vi "run.create.vi"(6 "Additional Configuration":T1, 8 "error in":errorcluster, 9 "Timing":cluster{"Start":timestamp, "End":timestamp} {"End" format="%<%x %.3X>T"; "Start" format="%<%x %.3X>T"}, 10 "Titles":cluster{"Name":string, "Description":string}, 11 "Nominal Client in":refnum<class "Nominal Client.lvclass">) -> (0 "error out":errorcluster, 2 "Run":refnum<class "Run.lvclass">, 3 "Nominal Client out":refnum<class "Nominal Client.lvclass">, 4 "Response body":string)   [LabVIEW 2020, in "Nominal Client.lvclass"]
doc: "Create a new run in Nominal.\nThrows if start is equal to or after end."
uses:
  Nominal Client.lvclass
  Run/Run.lvclass
  Nominal Client.lvclass/Nominal Client.ctl
  nominal types/workspace/workspace.lvclass/workspace.ctl
  workspace.get.vi
  <vilib>/JDP Science/JSONtext/Merge into Object.vi
  workspace.add_to_payload.vi/88650e10-de3e-481c-85db-71cb0fdf4485.vi
  nominal types/workspace/rid.get.vi
  <vilib>/LabVIEW Open Source Project/Epoch Date & Time/epoch.UNIX/Epoch.UNIX.lvclass
  C:/Program Files (x86)/National Instruments/LabVIEW 2020/vi.lib/LabVIEW Open Source Project/Epoch Date & Time/epoch/Epoch.lvclass
  <vilib>/LabVIEW Open Source Project/Epoch Date & Time/Get Epoch Time.vi
  <vilib>/JDP Science/JSONtext/Variant to JSON Text.vi
  <vilib>/JDP Science/JSONtext/Array of Variants to JSON Object.vi
  <vilib>/JDP Science/JSONtext/Set Item.vi
  <vilib>/JDP Science/JSONtext/Get all Object Items.vi
  <vilib>/JDP Science/JSONtext/Set Multiple Object Items.vi
  <vilib>/JDP Science/JSONtext/LVClass Serializer/JSONtext LVClass Serializer.lvclass
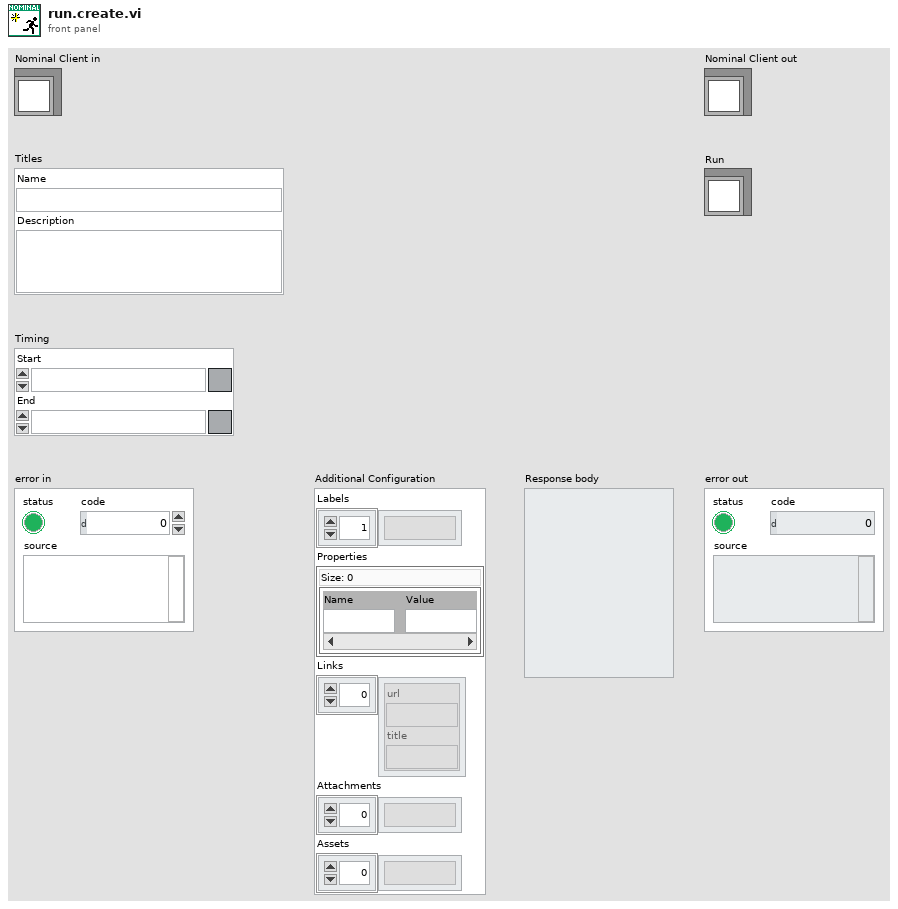
[diagram p1: front panel]
types:
  T1 = cluster{"Labels":string[], "Properties":map{string, string}, "Links":cluster{"url":string, "title":string}[], "Attachments":string[], "Assets":string[]}
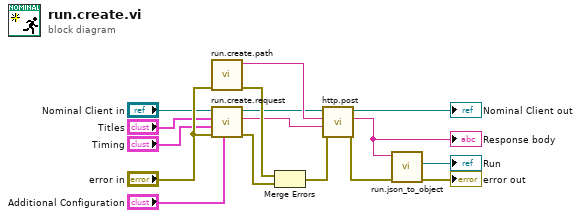
[diagram p0: block diagram]
diagram:
  n1 = call "run.create.path.vi"("error in"="error in") -> ("error out"=w5:errorcluster, "path"=w10:string)  [unwired: 9 in]
  n2 = call "run.create.request.vi"("Additional Configuration"="Additional Configuration", "error in (no error)"="error in", "Timing"="Timing", "Titles"="Titles", "Nominal Client in"="Nominal Client in") -> ("error out"=w4:errorcluster, "Request Body"=w1:string, "Nominal Client out"=w2:refnum<class "Nominal Client.lvclass">)  [unwired: 4 in]
  n3 = Merge Errors(w5, w4) -> (w3:errorcluster)
  n4 = call "http.post.vi"("error in"=w3, "Request body"=w1, "Path"=w10, "Nominal Client in"=w2) -> ("error out"=w13:errorcluster, "Response"=w14:string, "Nominal Client out"=→"Nominal Client out":refnum<class "Nominal Client.lvclass">)  [unwired: 4 in, 1 out]
  "Response body" <- w14
  n5 = call "run.json_to_object.vi"("error in"=w13, "JSON"=w14) -> ("error out"=→"error out":errorcluster, "Run"=→"Run":refnum<class "Run.lvclass">)  [unwired: 8 in]
